vi "ReadEncoders_v3.vi"(9 "PrevTick":u32, 10 "PrevPos":dbl[](array[numeric]), 11 "Reset Encoders":bool) -> (1 "Tick Count(uSec)":u32 caption="Tick Count(Ticks)", 2 "Speed":dbl[](array[numeric]), 3 "Pos":dbl[](array[numeric]))   [LabVIEW 2018]
uses:
  <vilib>/Studica/Studica Toolkit/Background/Mxp Selection.ctl
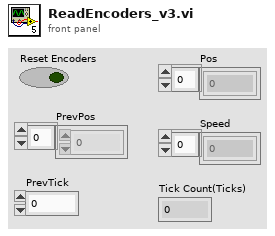
[diagram p1: front panel]
types:
  T1 = typedef "Mxp Selection.ctl" = enum16{"MXP A", "MXP B"}
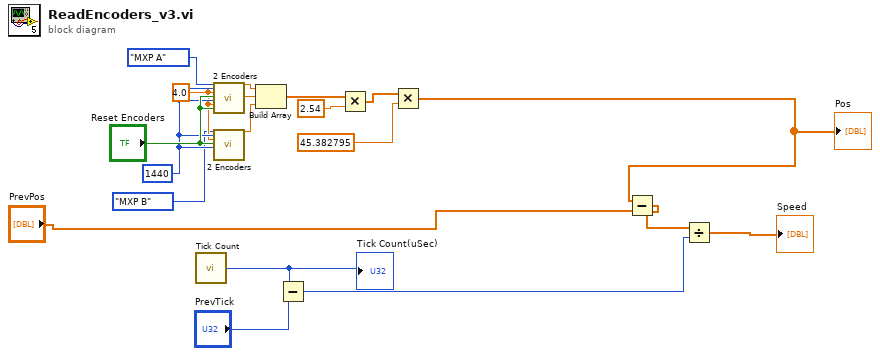
[diagram p0: block diagram]
diagram:
  w3 = 4.0 ("Wheel Diameter M1 (inches)")
  w4 = u32 1440 ("Ticks Per Rev M0")
  n1 = call "Tick Count"() -> ("Tick Count(uSec)"=w14:u32)
  "Tick Count(uSec)" <- w14
  n2 = call <vilib>:"2 Encoders.vi"("Mxp Side"=Mxp_Selection."MXP A", "Ticks Per Rev M0"=w4, "Wheel Diameter M0 (inches)"=w3, "Reset Encoder 0"="Reset Encoders", "Ticks Per Rev M1"=w4, "Wheel Diameter M1 (inches)"=w3, "Reset Encoder 1"="Reset Encoders") -> ("Distance M0 (inches)"=w6:dbl, "Distance M1 (inches)"=w7:dbl)  [unwired: 18 in, 1 out]
  n3 = call <vilib>:"2 Encoders.vi"("Mxp Side"=Mxp_Selection."MXP B", "Ticks Per Rev M0"=w4, "Wheel Diameter M0 (inches)"=w3, "Reset Encoder 0"="Reset Encoders", "Ticks Per Rev M1"=w4) -> ("Distance M0 (inches)"=w8:dbl)  [unwired: 20 in, 2 out]
  n4 = Build Array(w6, w7, w8) -> (w10:dbl[])
  n5 = Subtract(x=w14, y="PrevTick") -> (x-y=w16:u32)
  n6 = Multiply(x=w10, y=2.54) -> (x*y=w11:dbl[])
  n7 = Multiply(x=w11, y=45.382795) -> (x*y=w13:dbl[])
  "Pos" <- w13
  n8 = Subtract(x=w13, y="PrevPos") -> (x-y=w15:dbl[])
  n9 = Divide(x=w15, y=w16) -> (x/y=→"Speed":dbl[])
